vi "PWM_Heartbeat.vi"(3 "error in":errorcluster, 4 "Enable 2":bool, 5 "Enable":bool) -> (0 "error out":errorcluster)   [LabVIEW 2009, in "PWM.lvlib"]
doc: "Enables 2 PWM signals and sets them to default value (1,5 ms high, 20 ms period)."
uses:
  PWM.lvlib
  PWM_Name.ctl
panel:
  in  "PWM_in 2":T1=2 items=["Invalid"=0, "PWM1"=1, "PWM2"=2, "PWM9"=9, "PWM10"=10]
  in  "PWM_in":T1=1 items=["Invalid"=0, "PWM1"=1, "PWM2"=2, "PWM9"=9, "PWM10"=10]
  in  "Period (uSec)":u32=20000
  in  "High (uSec)":u32=1500
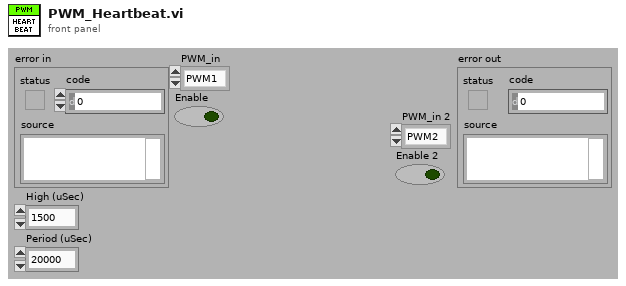
[diagram p1: front panel]
types:
  T1 = typedef "PWM.lvlib/PWM_Name.ctl" = u16
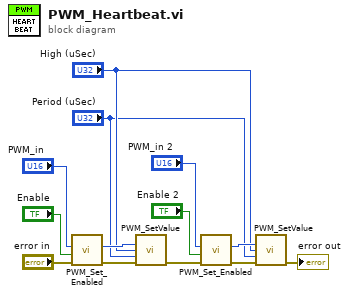
[diagram p0: block diagram]
diagram:
  n1 = call "PWM_Set_Enabled.vi"("error in"="error in", "Enable"="Enable", "PWM_in"="PWM_in") -> ("error out"=w13:errorcluster, "PWM_out"=w11:T1)  [unwired: 7 in]
  n2 = call "PWM_SetValue.vi"("PWM"=w11, "High (uSec)"="High (uSec)", "Period (uSec)"="Period (uSec)", "error in"=w13) -> ("error out"=w4:errorcluster)  [unwired: 11 in]
  n3 = call "PWM_Set_Enabled.vi"("error in"=w4, "Enable"="Enable 2", "PWM_in"="PWM_in 2") -> ("error out"=w8:errorcluster, "PWM_out"=w7:T1)  [unwired: 7 in]
  n4 = call "PWM_SetValue.vi"("PWM"=w7, "High (uSec)"="High (uSec)", "Period (uSec)"="Period (uSec)", "error in"=w8) -> ("error out"=→"error out":errorcluster)  [unwired: 11 in]
